vi "Surface Force Set.vi"(8 "error in (no error)":errorcluster, 9 "Force Constants":cluster{"k1":dbl, "k2":dbl, "k3":dbl, "k4":dbl}={"k1"=1.0, "k2"=1.0, "k3"=1.0, "k4"=1.0}, 10 "Force Settings":u16(ring) items=["0", "1", "2", "3", "4"]) -> (0 "error out":errorcluster)   [LabVIEW 2017, in "Haptic Prog Interface.lvlib"]
doc: "Returns the horizontal xy-position of the haptic pen in nm, and the vertical z-position in mm. The horizontal position depends on the frame origin and frame size.\n\n<b>Position:</b> Returns a cluster of the x (nm), y (nm), and z (mm) positions of the pen."
uses:
  Haptic Prog Interface.lvlib
  Haptic-Programming-Interface/src/x64/Debug/Haptic Programming Interface.dll
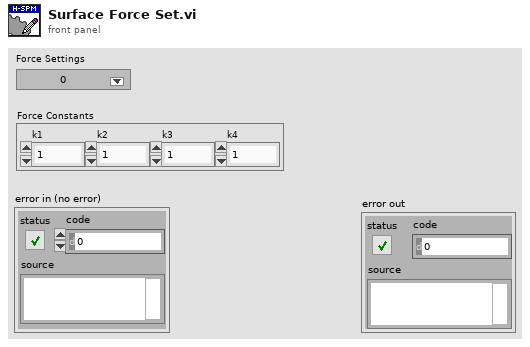
[diagram p1: front panel]
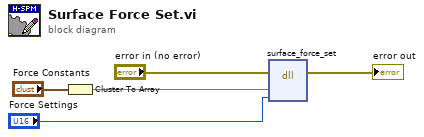
[diagram p0: block diagram]
diagram:
  n1 = Cluster To Array(cluster="Force Constants") -> (array=w2:dbl[])
  n2 = dll-call lib="C:/Users/freem/Documents/GitHub/HapticSPM/Haptic-Programming-Interface/src/x64/Debug/Haptic Programming Interface.dll" fn="surface_force_set"(error in="error in (no error)", "input"=w2, "setting"="Force Settings") -> (error out=→"error out":errorcluster)  [unwired: 5 in, 1 out]
